vi "Read ConvBox Handler.vi"(8 "error in (no error)":errorcluster, 11 "Listener in":refnum<class "Listener.lvclass">) -> (0 "error out":errorcluster, 3 "Listener out":refnum<class "Listener.lvclass">)   [LabVIEW 2019, in "Listener.lvclass"]
uses:
  Listener.lvclass
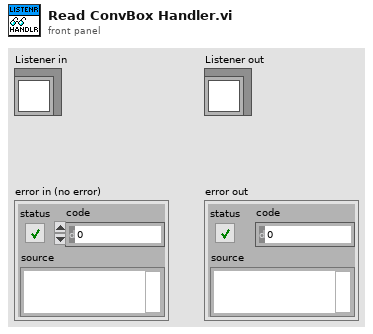
[diagram p1: front panel]
types:
  T1 = typedef "Listener.lvclass/RS-xxx To GPIB ConvBox Data Structure.ctl" = cluster{"Protocol Port Ref":refnum<visa-resource-name>, "Listener Port Ref":refnum<visa-resource-name>, "Data":string, "Command Messages Read":string[], "Address":string}
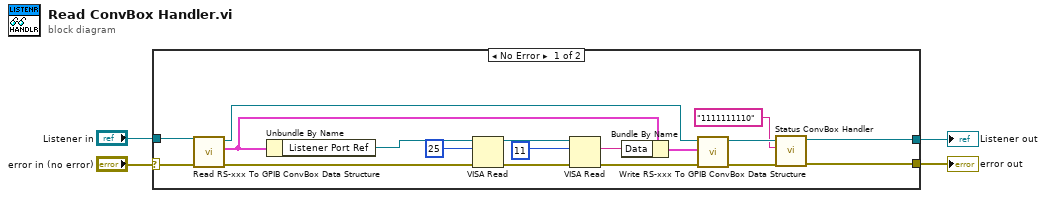
[diagram p0: block diagram]
diagram:
  n1 = case shown="No Error" "error in (no error)" {
    selector: "error in (no error)" -> [w18 w23]
    tunnel: "Listener in" -> [w17 w24]
    tunnel: [w6 w23] -> w2
    tunnel: [w5 w24] -> w1
    frame No Error {
      n2 = call-dynamic "Read RS-xxx To GPIB ConvBox Data Structure.vi"("error in (no error)"=w18, "Listener in"=w17) -> ("error out"=w16:errorcluster, "RS-xxx To GPIB ConvBox Data Structure"=w14:T1, "Listener out"=w9:refnum<class "Listener.lvclass">)  [unwired: 7 in]
      n3 = Unbundle By Name(w14) -> ("Listener Port Ref"=w15:refnum<visa-resource-name>)
      n4 = VISA Read(VISA resource name=w15, byte count=u32 25, error in (no error)=w16) -> (VISA resource name out=w21:refnum<visa-resource-name>, error out=w20:errorcluster)  [unwired: 2 out]
      n5 = VISA Read(VISA resource name=w21, byte count=u32 11, error in (no error)=w20) -> (read buffer=w13:string, error out=w12:errorcluster)  [unwired: 2 out]
      n6 = Bundle By Name(cluster=w14, "Data"=w13) -> (w10:T1)
      n7 = call-dynamic "Write RS-xxx To GPIB ConvBox Data Structure.vi"("error in (no error)"=w12, "RS-xxx To GPIB ConvBox Data Structure"=w10, "Listener in"=w9) -> ("error out"=w11:errorcluster, "Listener out"=w8:refnum<class "Listener.lvclass">)  [unwired: 7 in]
      n8 = call "Status ConvBox Handler.vi"("error in(no error)"=w11, "Value In"="1111111110" ("write buffer"), "Listener in"=w8) -> ("error out"=w6:errorcluster, "Listener out"=w5:refnum<class "Listener.lvclass">)  [unwired: 7 in]
    }
    frame Error {
    }
  }
  "error out" <- w2
  "Listener out" <- w1
